vi "test Acyclic Loopback Value Overflow.vi"(8 "error in":errorcluster, 11 "TestCase in":refnum<class "Single Board 1Ch Loopback.lvclass">) -> (0 "error out":errorcluster, 3 "TestCase out":refnum<class "Single Board 1Ch Loopback.lvclass">)   [LabVIEW 2020, in "Single Board 1Ch Loopback.lvclass"]
uses:
  Single Board 1Ch Loopback.lvclass
  C:/dev/git/niveristand-custom-device-testing-tools/VeriStandTestCase/VeriStandTestCase.lvclass
  <vilib>/numeric/Random Number (Range) U64.vi
  <vilib>/numeric/sub_Random U32.vi
  <vilib>/NI VeriStand/Execution/Workspace/NI VeriStand - Set Multiple Channel Values.vi
  <vilib>/addons/_JKI Toolkits/VI Tester/TestCase.llb/TestCase.lvclass
  <vilib>/NI VeriStand/Execution/Workspace/NI_VS Workspace ExecutionAPI.lvlib
  niveristand-custom-device-testing-tools/VeriStandTestUtilities/VeriStandTestUtilities.lvlib
  C:/Program Files (x86)/National Instruments/LabVIEW 2020/vi.lib/addons/_JKI Toolkits/VI Tester/TestCase.llb/TestCase.lvclass
  C:/dev/git/niveristand-aim-arinc429-custom-device/Source/Custom Device Support/Tests/System/Single Board (CH2--CH3) Loopback/Single Board 1Ch Loopback.lvclass
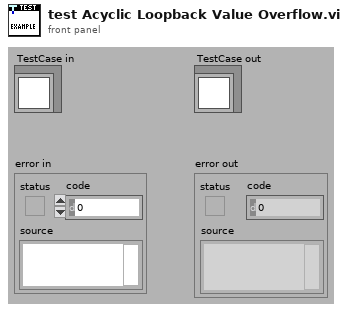
[diagram p1: front panel]
types:
  T1 = typedef "NI_VS Workspace ExecutionAPI.lvlib/WorkspaceAPI.ctl" = refnum<k24>
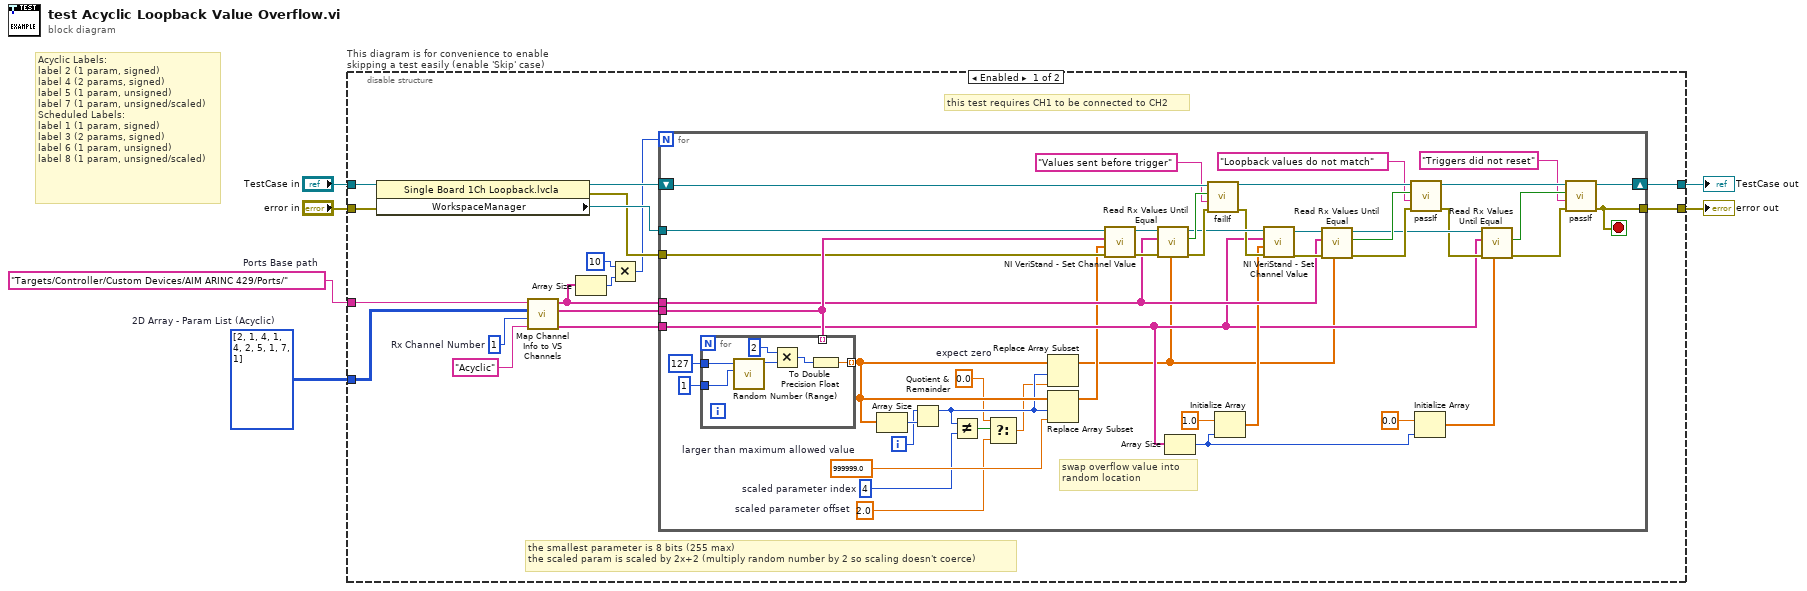
[diagram p0: block diagram]
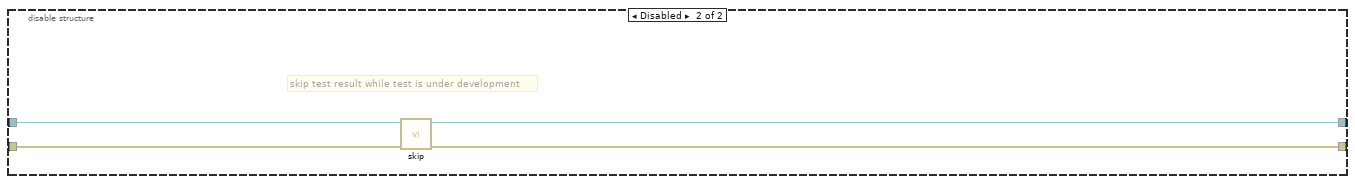
[diagram p2: hidden frame]
diagram:
  w2 = i32[][] [[2, 1], [4, 1], [4, 2], [5, 1], [7, 1]]  # 2D Array - Param List (Acyclic)
  w3 = "Targets/Controller/Custom Devices/AIM ARINC 429/Ports/"  # Ports Base path
  # "Acyclic Labels:\nlabel 2 (1 param, signed)\nlabel 4 (2 params, signed)\nlabel 5 (1 param, unsigned)\nlabel 7 (1 param, unsigned/scaled)\nScheduled Labels:\nlabel 1 (1 param, signed)\nlabel 3 (2 params, signed)\nlabel 6 (1 param, unsigned)\nlabel 8 (1 param, unsigned/scaled)"
  n1 = disable-structure "This diagram is for convenience to enable skipping a test easily (enable 'Skip' case)" shown="Enabled" {
    disable-tunnel: "TestCase in" -> [w19 w79]
    disable-tunnel: [w17 w77] -> w1
    disable-tunnel: [w16 w78] -> w5
    disable-tunnel: "error in" -> [w18 w76]
    disable-tunnel: w3 -> [w20 _]
    disable-tunnel: w2 -> [w13 _]
    frame Enabled {
      w14 = 1  # Rx Channel Number
      # "this test requires CH1 to be connected to CH2"
      # "the smallest parameter is 8 bits (255 max)\nthe scaled param is scaled by 2x+2 (multiply random number by 2 so scaling doesn't coerce)"
      n2 = property class="Single Board 1Ch Loopback.lvcla"(reference=w19, error in=w18) -> (reference out=w21:refnum<class "Single Board 1Ch Loopback.lvclass">, error out=w22:errorcluster, "WorkspaceManager"=w23:T1)
      n3 = call "Map Channel Info to VS Channels.vi"("Transfer Type"="Acyclic", "Rx Channel Number"=w14, "2D Array - Label/Param List"=w13, "VS Channel Base Port"=w20) -> ("Tx Trigger Channels Array"=w11:string[], "Tx Channels Array"=w12:string[], "Rx Channels Array"=w8:string[])  [unwired: 4 in, 1 out]
      n4 = Array Size(array=w8) -> (size(s)=w9:i32)
      n5 = Multiply(x=10, y=w9) -> (x*y=w7:i32)
      n6 = for {
        N: w7 -> [_]
        tunnel: w8 -> [w55]
        tunnel: w23 -> [w67]
        tunnel: w22 -> [w60]
        tunnel: w12 -> [w66]
        shift-right: [w49] -> w17
        shift-left: w21 -> [w62]
        tunnel: [w51] -> w16
        tunnel: w11 -> [w39]
        i -> [w30]
        stop <- w51 stop-if-true
        w26 = 2.0  # scaled parameter offset
        w27 = 4  # scaled parameter index
        w25 = 0.0  # expect zero
        w34 = 999999.0  # larger than maximum allowed value
        # "swap overflow value into \nrandom location"
        n7 = for {
          tunnel: [w74] -> w31 mode=indexing
          tunnel: u64 127 ("upper bound (100)") -> [w73]
          tunnel: u64 1 ("upper bound (100)") -> [w72]
          tunnel: w66 -> [_] mode=indexing
          n8 = call-poly <vilib>:"Random Number (Range).vi"("lower bound (0)"=w72, "upper bound (100)"=w73) -> ("number"=w75:u64)  [unwired: 9 in]
          n9 = Multiply(x=u64 2, y=w75) -> (x*y=w71:u64)
          n10 = To Double Precision Float(number=w71) -> (double precision float=w74:dbl)
        }
        n11 = Array Size(array=w31) -> (size(s)=w32:i32)
        n12 = Quotient & Remainder(x=w30, y=w32) -> (x-y*floor(x/y)=w28:i32)  [unwired: 1 out]
        n13 = Not Equal?(x=w28, y=w27) -> (x != y?=w29:bool)
        n14 = Select(t=w25, s=w29, f=w26) -> (s? t:f=w24:dbl)
        n15 = Replace Array Subset(array=w31, new element=w24, index=w28) -> (w33:dbl[])
        n16 = Replace Array Subset(array=w31, new element=w34, index=w28) -> (w35:dbl[])
        n17 = call-poly <vilib>:"NI VeriStand - Set Channel Value.vi"("error in (no error)"=w60, "Values"=w35, "Channels"=w66, "WorkspaceManager in"=w67) -> ("error out"=w63:errorcluster, "WorkspaceManager out"=w65:T1)  [unwired: 6 in]
        n18 = call "Read Rx Values Until Equal.vi"("expected values"=w33, "error in"=w63, "Rx aliases"=w55, "workspace manager in"=w65) -> ("error out"=w64:errorcluster, "values equal expected"=w61:bool, "workspace manager out"=w59:T1)  [unwired: 5 in]
        n19 = Array Size(array=w39) -> (size(s)=w36:i32)
        n20 = call-dynamic "failIf.vi"("error in (no error)"=w64, "message (\"\")"="Values sent before trigger" ("message (\"\")"), "fail"=w61, "TestCase in"=w62) -> ("error out"=w58:errorcluster, "TestCase out"=w52:refnum<class "Single Board 1Ch Loopback.lvclass">)  [unwired: 6 in]
        n21 = Initialize Array(1.0, w36) -> (w40:dbl[])
        n22 = call-poly <vilib>:"NI VeriStand - Set Channel Value.vi"("error in (no error)"=w58, "Values"=w40, "Channels"=w39, "WorkspaceManager in"=w59) -> ("error out"=w56:errorcluster, "WorkspaceManager out"=w57:T1)  [unwired: 6 in]
        n23 = call "Read Rx Values Until Equal.vi"("expected values"=w33, "error in"=w56, "Rx aliases"=w55, "workspace manager in"=w57) -> ("error out"=w53:errorcluster, "values equal expected"=w54:bool, "workspace manager out"=w47:T1)  [unwired: 5 in]
        n24 = call-dynamic "passIf.vi"("error in (no error)"=w53, "message (\"\")"="Loopback values do not match" ("message (\"\")"), "pass"=w54, "TestCase in"=w52) -> ("error out"=w46:errorcluster, "TestCase out"=w50:refnum<class "Single Board 1Ch Loopback.lvclass">)  [unwired: 6 in]
        n25 = Initialize Array(0.0, w36) -> (w37:dbl[])
        n26 = call "Read Rx Values Until Equal.vi"("expected values"=w37, "error in"=w46, "Rx aliases"=w39, "workspace manager in"=w47) -> ("error out"=w45:errorcluster, "values equal expected"=w48:bool)  [unwired: 5 in, 1 out]
        n27 = call-dynamic "passIf.vi"("error in (no error)"=w45, "message (\"\")"="Triggers did not reset" ("message (\"\")"), "pass"=w48, "TestCase in"=w50) -> ("error out"=w51:errorcluster, "TestCase out"=w49:refnum<class "Single Board 1Ch Loopback.lvclass">)  [unwired: 6 in]
      }
    }
    frame Disabled {
      # "skip test result while test is under development"
      n28 = call <vilib>:"skip.vi"("error in (no error)"=w76, "TestCase in"=w79) -> ("error out"=w78:errorcluster, "TestCase out"=w77:refnum<class "Single Board 1Ch Loopback.lvclass">)  [unwired: 8 in]
    }
  }
  "error out" <- w5
  "TestCase out" <- w1
